vi "Run_Close Core.vi"(0 "functionbase in":refnum<class "functionbase.lvclass">, 11 "error in (no error)":errorcluster) -> (4 "functionbase out":refnum<class "functionbase.lvclass">, 15 "error out":errorcluster)   [LabVIEW 2019, in "LSL.lvlib" / "functionbase.lvclass"]
uses:
  functionbase.lvclass
  functionbase.lvclass/functionbase.ctl
  properties/Read RT Variables.vi
  properties/Read Indent#.vi
  variables/RT Variables/RT Variables.lvclass
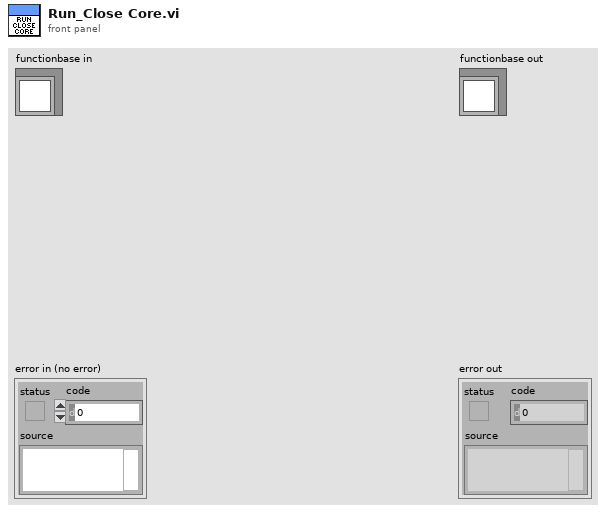
[diagram p1: front panel]
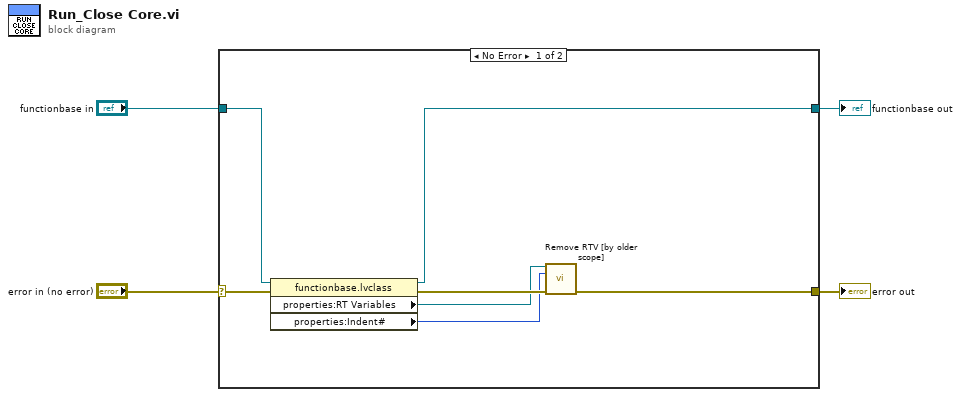
[diagram p0: block diagram]
diagram:
  n1 = case shown="No Error" "error in (no error)" {
    selector: "error in (no error)" -> [w9 w13]
    tunnel: [w7 w13] -> w3
    tunnel: [w10 w12] -> w1
    tunnel: "functionbase in" -> [w11 w12]
    frame No Error {
      n2 = property class="functionbase.lvclass"(reference=w11, error in=w9) -> (reference out=w10:refnum<class "functionbase.lvclass">, error out=w8:errorcluster, "properties:RT Variables"=w5:refnum<class "RT Variables.lvclass">, "properties:Indent#"=w6:i64)
      n3 = call-dynamic "Remove RTV [by older scope].vi"("RT Variables in"=w5, "RTV Scope"=w6, "error in (no error)"=w8) -> ("error out"=w7:errorcluster)  [unwired: 11 in, 1 out]
    }
    frame Error {
    }
  }
  "error out" <- w3
  "functionbase out" <- w1
